vi "manual_test_coag_dose.vi"(10 "Enum":T2=enum."Target") -> ()   [LabVIEW 2019]
uses:
  enum_observed_clarified.ctl
  RowData_Type.ctl
  give_data_NR.ctl
  <vilib>/gmath/zero.llb/Newton Raphson Zero Finder (VI).vi
  <vilib>/gmath/NI_Gmath.lvlib
panel:
  out "Coag_dose":dbl
  in  "RowData":T1
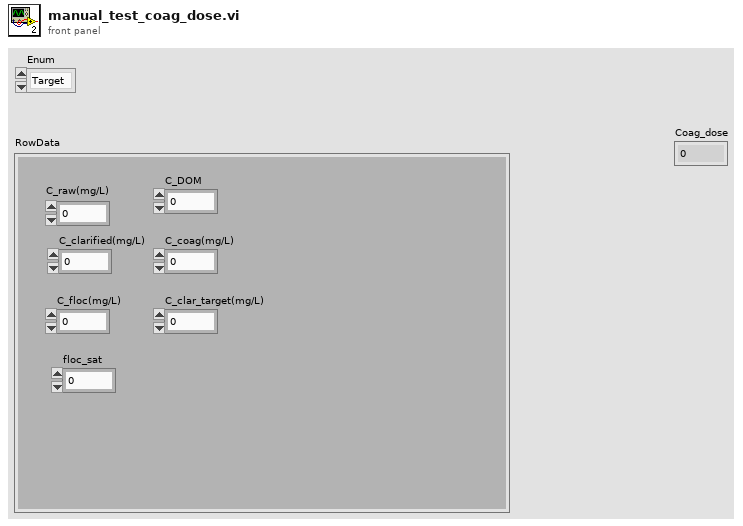
[diagram p1: front panel]
types:
  T1 = typedef "RowData_Type.ctl" = cluster{"C_raw(mg/L)":dbl, "C_clarified(mg/L)":dbl, "C_floc(mg/L)":dbl, "floc_sat":dbl, "C_DOM":dbl, "C_coag(mg/L)":dbl, "C_clar_target(mg/L)":dbl}
  T2 = typedef "enum_observed_clarified.ctl" = enum16{"Observed", "Target"}
  T3 = typedef "give_data_NR.ctl" = cluster{"RowData":T1, "Enum":T2}
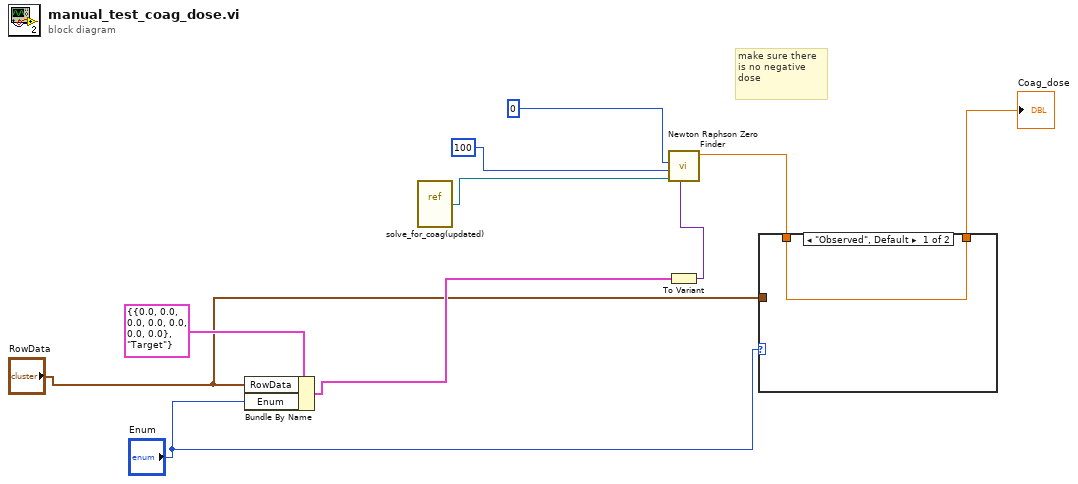
[diagram p0: block diagram]
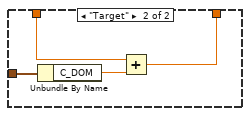
[diagram p2: hidden frame]
diagram:
  # "make sure there is no negative dose"
  n1 = Bundle By Name(cluster=T3 {"RowData"={"C_raw(mg/L)"=0.0, "C_clarified(mg/L)"=0.0, "C_floc(mg/L)"=0.0, "floc_sat"=0.0, "C_DOM"=0.0, "C_coag(mg/L)"=0.0, "C_clar_target(mg/L)"=0.0}, "Enum"=enum."Target"} ("data to NR"), "RowData"="RowData", "Enum"="Enum") -> (w5:T3)
  n2 = vi-ref "solve_for_coag(updated).vi"() -> (w8:refnum<vi>)
  n3 = To Variant(anything=w5) -> (Variant=w7:variant)
  n4 = call-poly <vilib>:"Newton Raphson Zero Finder.vi"("data"=w7, "f(x)"=w8, "end"=100, "start"=0) -> ("zero"=w2:dbl)  [unwired: 4 in, 3 out]
  n5 = case shown="\"Observed\", Default" "Enum" {
    tunnel: "RowData" -> [_ w15]
    tunnel: w2 -> [w11 w13]
    tunnel: [w11 w12] -> w1
    frame "Observed", Default {
    }
    frame "Target" {
      n6 = Unbundle By Name(w15) -> ("C_DOM"=w14:dbl)
      n7 = Add(x=w13, y=w14) -> (x+y=w12:dbl)
    }
  }
  "Coag_dose" <- w1
